vi "Append.vi"(8 "error in (no error)":errorcluster, 10 "SensorData in 2":refnum<class "SensorData.lvclass">, 11 "Double Scalar SensorData in":refnum<class "Double Scalar SensorData.lvclass">) -> (0 "error out":errorcluster, 3 "Double Scalar SensorData out":refnum<class "Double Scalar SensorData.lvclass">)   [LabVIEW 2012, in "Sensor Definition.lvlib" / "Double Scalar SensorData.lvclass"]
uses:
  Double Scalar SensorData.lvclass
  SensorData.lvclass
  Double Scalar SensorData.lvclass/Double Scalar SensorData.ctl
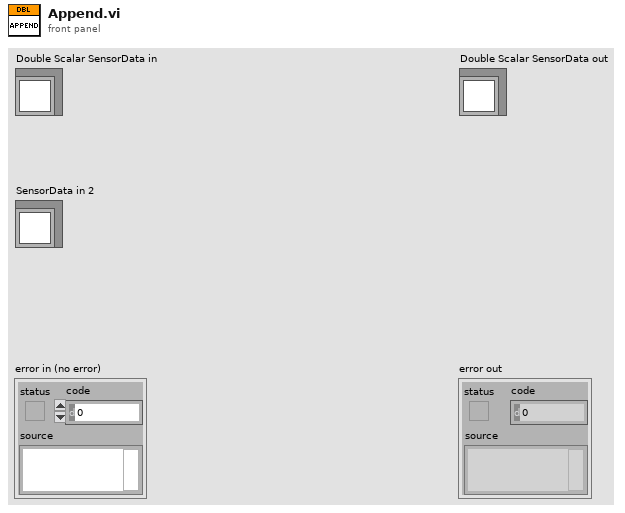
[diagram p1: front panel]
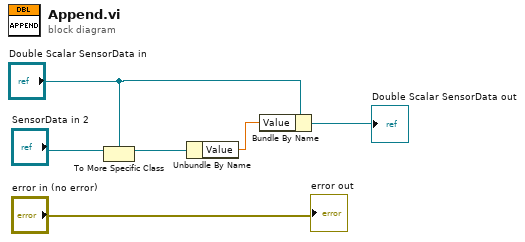
[diagram p0: block diagram]
diagram:
  n1 = To More Specific Class(target class="Double Scalar SensorData in", reference="SensorData in 2") -> (specific class reference=w5:refnum<class "Double Scalar SensorData.lvclass">)  [unwired: 1 in, 1 out]
  n2 = Unbundle By Name(w5) -> ("Value"=w3:dbl)
  n3 = Bundle By Name(cluster="Double Scalar SensorData in", "Value"=w3) -> (→"Double Scalar SensorData out":refnum<class "Double Scalar SensorData.lvclass">)
  "error out" <- "error in (no error)"
